vi "Principal.vi"() -> ()   [LabVIEW 2020]
panel:
  in  "Conversor Dis":bool
  in  "stop":bool
  in  "Conversor Grad":bool
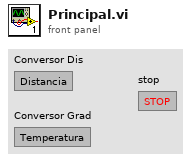
[diagram p1: front panel]
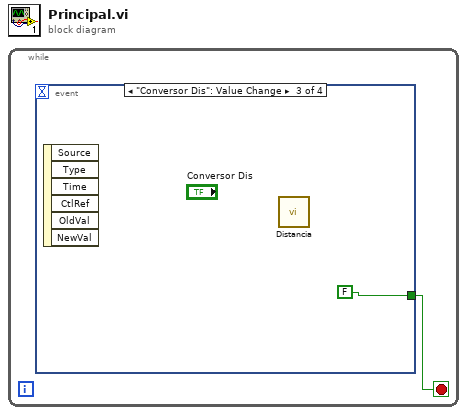
[diagram p0: block diagram]
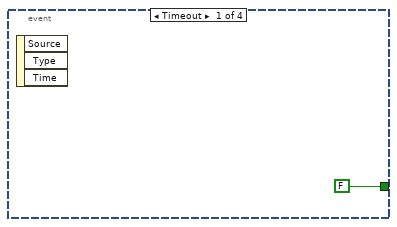
[diagram p2: hidden frame]
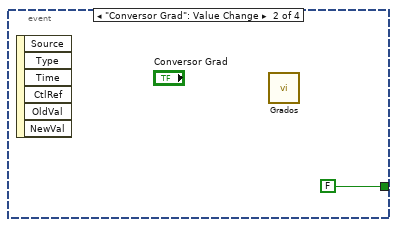
[diagram p3: hidden frame]
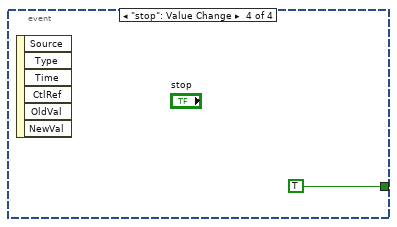
[diagram p4: hidden frame]
diagram:
  n1 = while {
    stop <- w1 stop-if-true
    n2 = event shown="[2] \"Conversor Dis\": Value Change" {
      selector: _ -> [_ _ _ _]
      dyn-events: _ -> [_ _ _ _]
      timeout: _ -> [_ _ _ _]
      tunnel: [FALSE FALSE FALSE TRUE] -> w1
      event Timeout {
        n3 = event-data() -> ()  [unwired: 1 in, 3 out]
      }
      event "Conversor Grad": Value Change {
        n4 = event-data() -> ()  [unwired: 1 in, 6 out]
        n5 = call "Grados.vi"() -> ()  [unwired: 4 in, 4 out]
      }
      event "Conversor Dis": Value Change {
        n6 = event-data() -> ()  [unwired: 1 in, 6 out]
        n7 = call "Distancia.vi"() -> ()  [unwired: 4 in, 4 out]
      }
      event "stop": Value Change {
        n8 = event-data() -> ()  [unwired: 1 in, 6 out]
      }
    }
  }
